vi "Read Timeout (ms).vi"(8 "error in (no error)":errorcluster, 11 "Wait On Integer Step in":refnum<class "Wait On Integer.lvclass">) -> (0 "error out":errorcluster, 2 "Timeout (ms)":i32, 3 "Wait On Integer Step out":refnum<class "Wait On Integer.lvclass">)   [LabVIEW 2018, in "Wait On Integer.lvclass"]
uses:
  Wait On Integer.lvclass
  Wait On Integer.lvclass/Wait On Integer.ctl
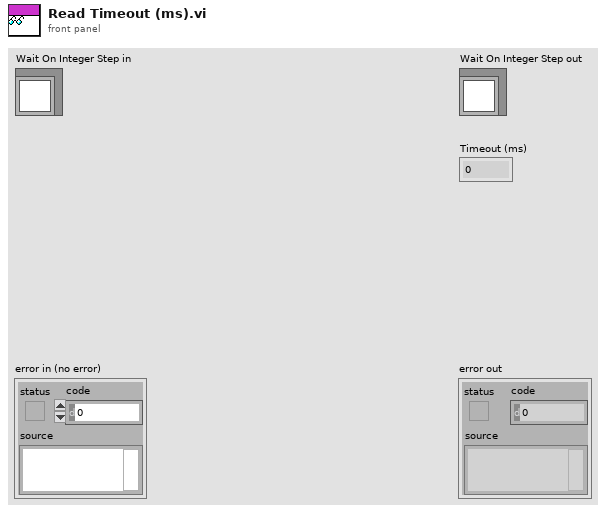
[diagram p1: front panel]
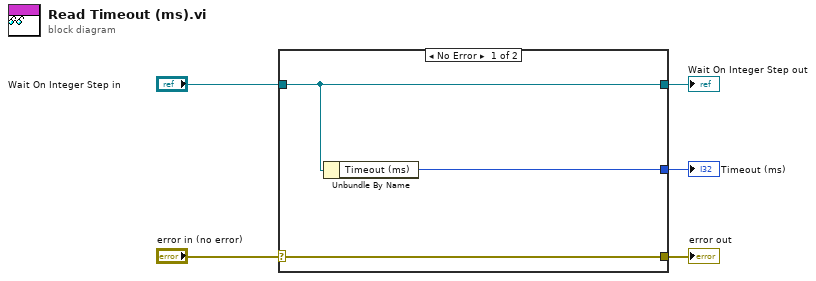
[diagram p0: block diagram]
diagram:
  n1 = case shown="No Error" "error in (no error)" {
    selector: "error in (no error)" -> [w8 w9]
    tunnel: [w8 w9] -> w4
    tunnel: [w7 w10] -> w2
    tunnel: "Wait On Integer Step in" -> [w7 w10]
    tunnel: [w6 _] -> w1
    frame No Error {
      n2 = Unbundle By Name(w7) -> ("Timeout (ms)"=w6:i32)
    }
    frame Error {
    }
  }
  "error out" <- w4
  "Wait On Integer Step out" <- w2
  "Timeout (ms)" <- w1
